vi "Main.vi"() -> ()   [LabVIEW 2020]
uses:
  <vilib>/userDefined/High Color/IMAQdx.ctl
  <vilib>/vision/Image Controls.llb/IMAQ Image.ctl
  <vilib>/DAQmx/write.llb/DAQmx Write (Analog Wfm 1Chan NSamp).vi
  <vilib>/Utility/error.llb/Error Cluster From Error Code.vi
  <vilib>/DAQmx/miscellaneous.llb/DAQmx Fill In Error Info.vi
  <vilib>/ErrorRing/Error Ring.xnode
  SuportVI2/Message Queue/Message Queue.lvlib
  SuportVI2/User Event - Stop/User Event - Stop.lvlib
  <vilib>/vision/driver/NI_Vision_Acquisition_Software.lvlib
  <vilib>/Analysis/NI_AALBase.lvlib
panel:
  in  "Generator Configuration":T1
  out "Image":T2(plugin-control)
  in  "Camera Config":cluster{"Camera Select":T3}
  in  "Exit":bool
  in  "Stop Camera":bool
  in  "Start Camera":bool
  out "Status Line":string
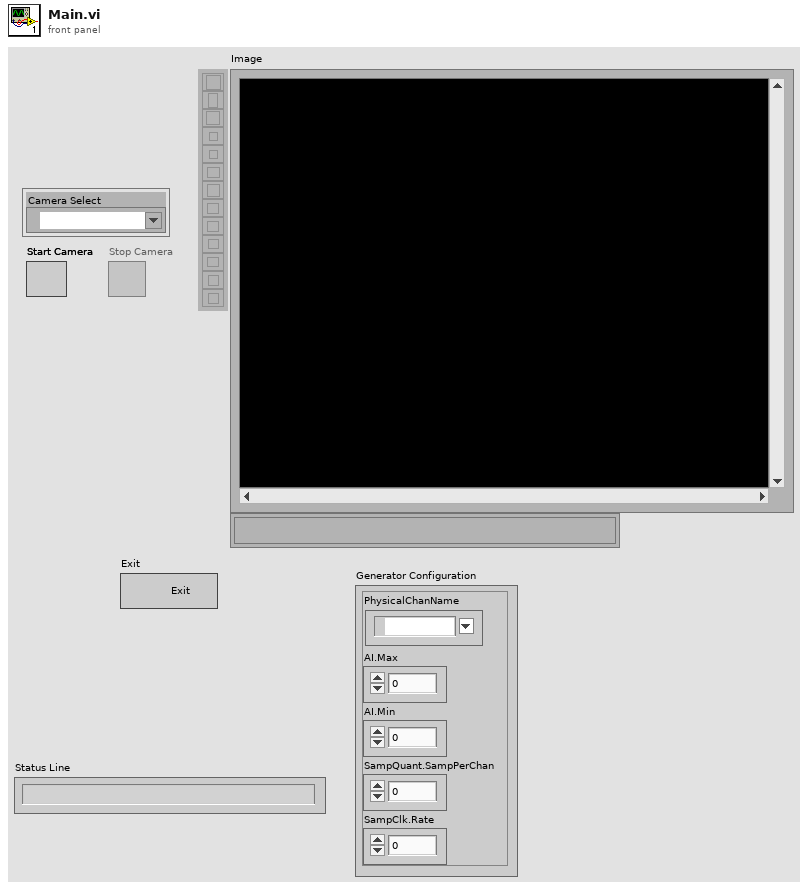
[diagram p1: front panel]
types:
  T1 = cluster{"SampClk.Rate":dbl, "SampQuant.SampPerChan":i32, "AI.Min":dbl, "AI.Max":dbl, "PhysicalChanName":tag}
  T2 = typedef "IMAQ Image.ctl" = refnum<image>
  T3 = typedef "IMAQdx.ctl" = refnum<k21>
  T4 = cluster{"DAQmx Task":refnum<k21>, "DAQmx Chanel":cluster{"SampClk.Rate":dbl, "SampQuant.SampPerChan":i32, "AI.Min":dbl, "AI.Max":dbl, "PhysicalChanName":tag}, "DB Data":dbl[][]}
  T5 = cluster{"Image":cluster{"Image original":T2, "Image copy":T2, "Image Out":T2}, "Session Config":cluster{"Session":T3}, "Data":string}
  T6 = cluster{"Start Camera":refnum<vi>, "Stop Camera":refnum<vi>, "Exit":refnum<vi>, "Camera Conf":refnum<vi>, "Status Line":refnum<vi>, "Status Line Text":string, "Camera Select":refnum<vi>}
  T7 = cluster{"UI":refnum<queue>, "Camera":refnum<queue>, "Acquire":refnum<queue>, "SinusGen":refnum<queue>}
  T8 = typedef "Image Type" = u32
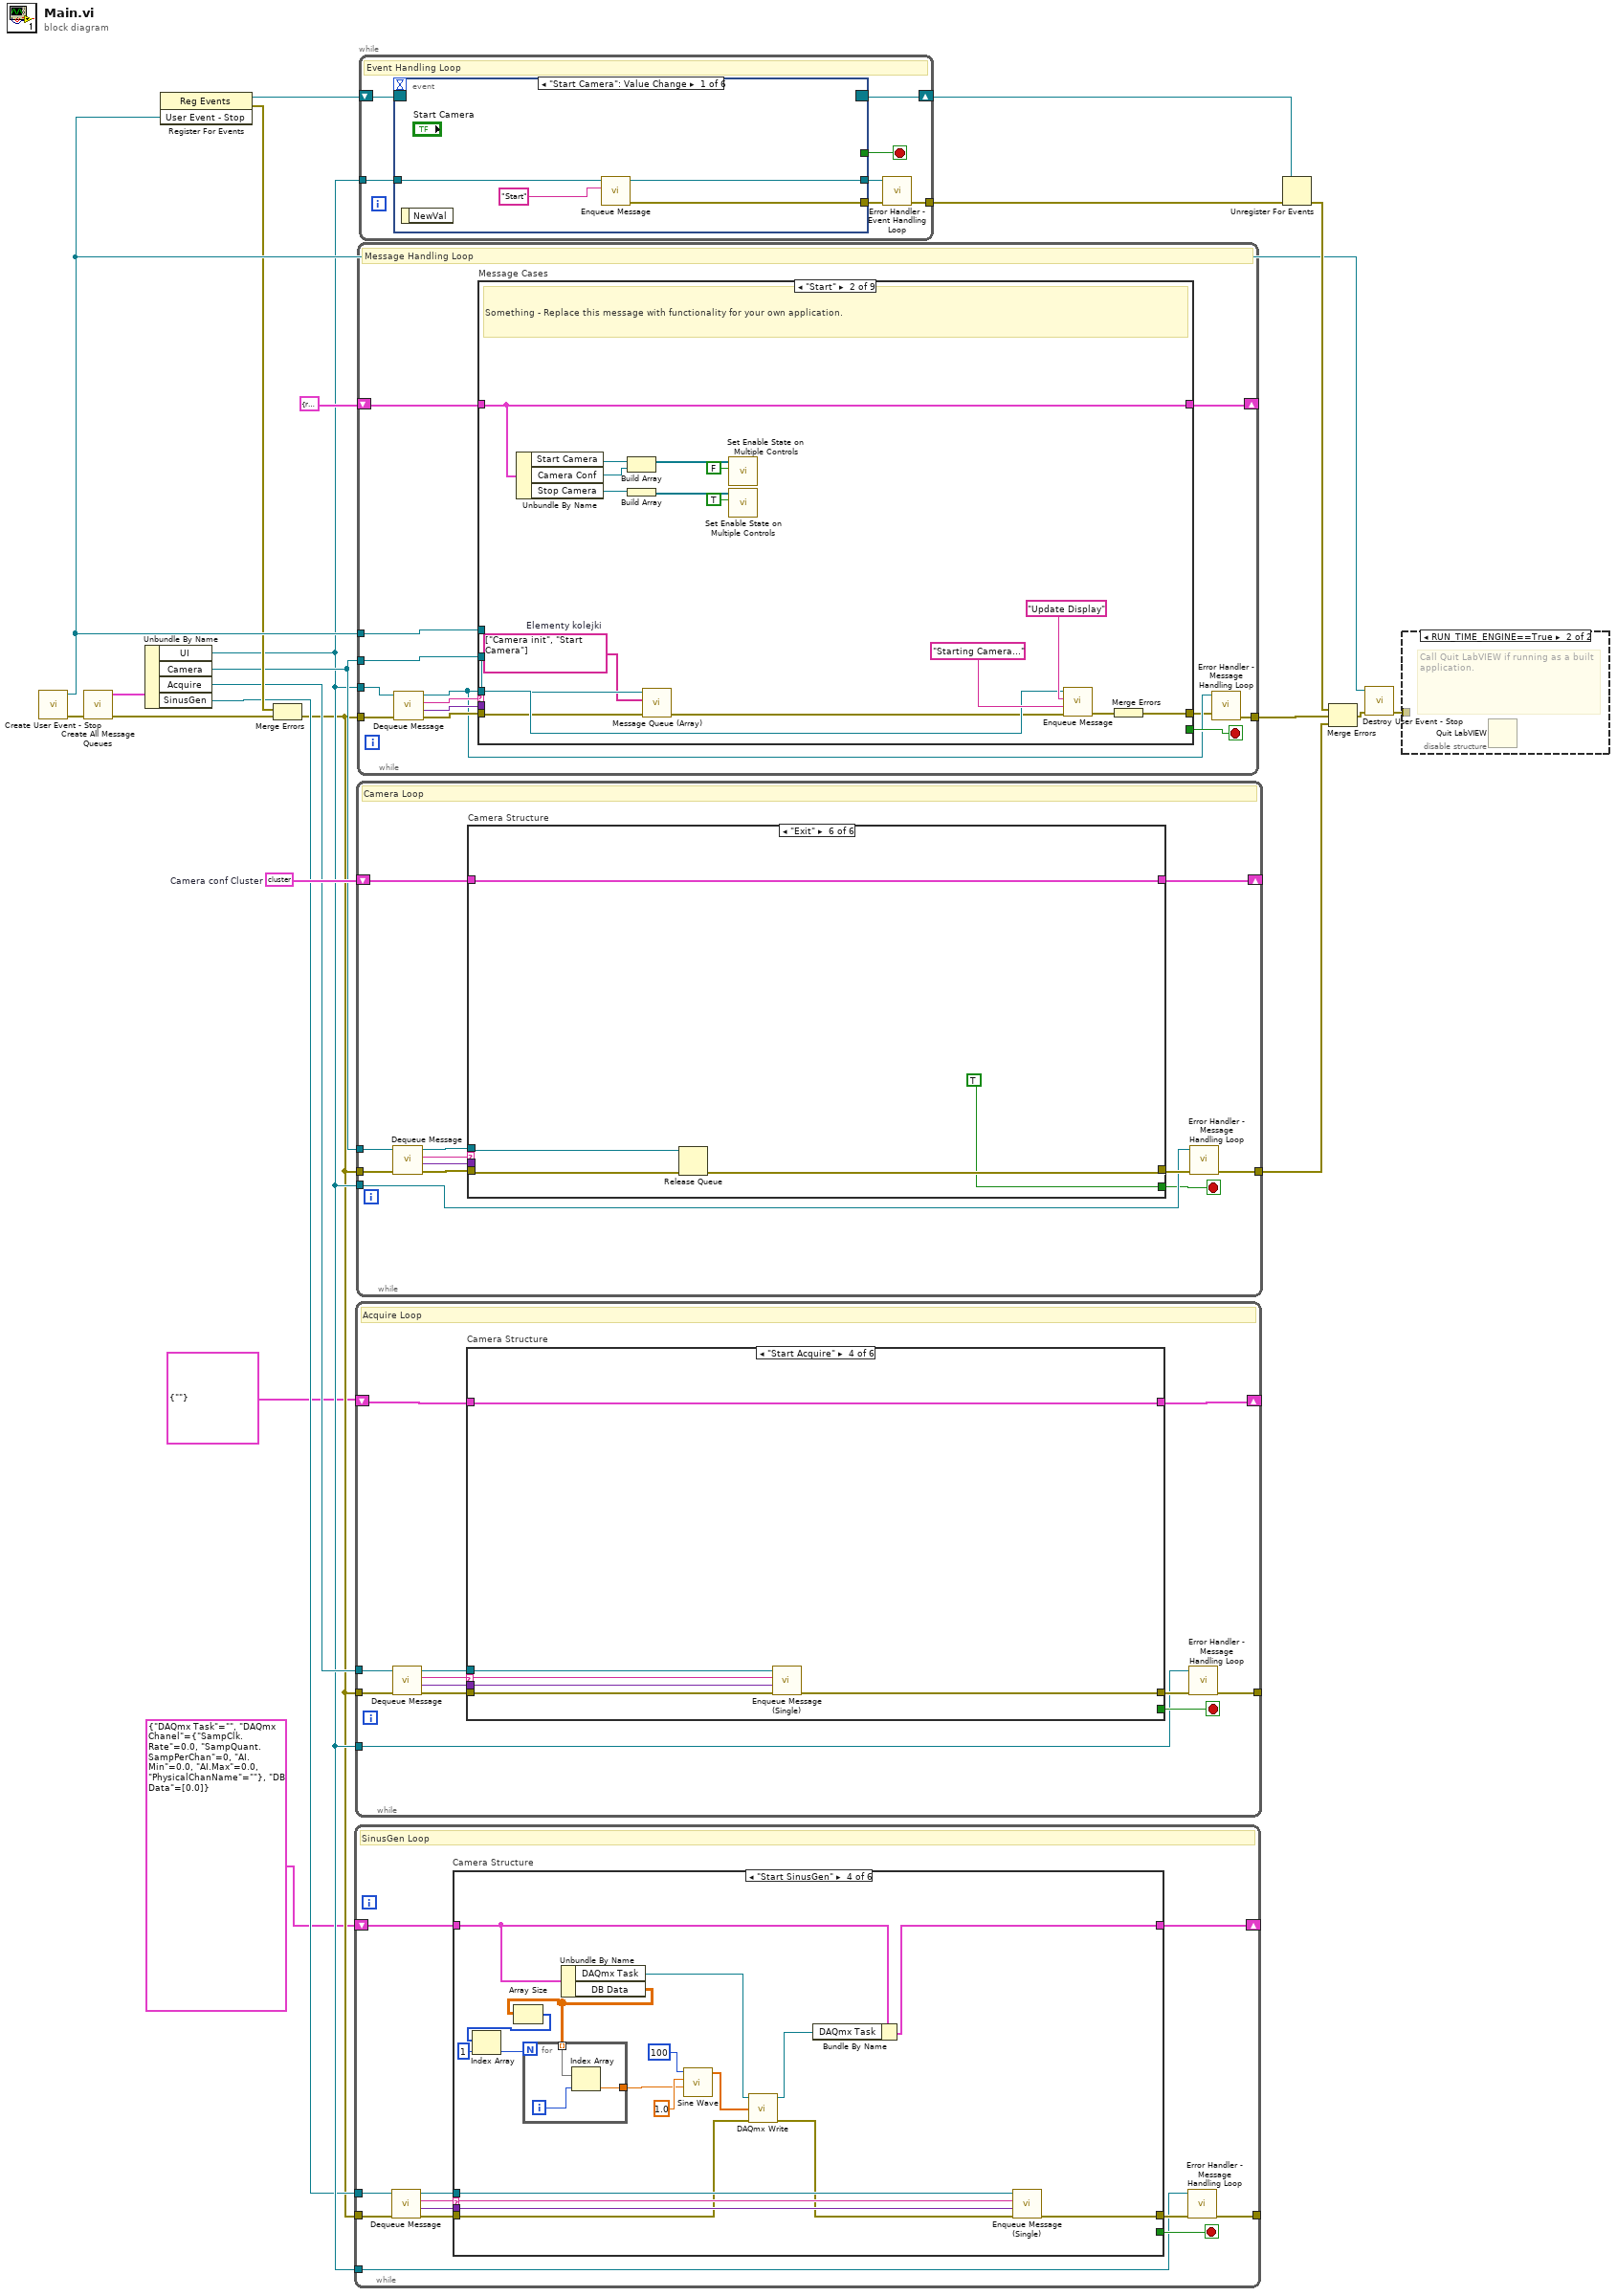
[diagram p0: block diagram]
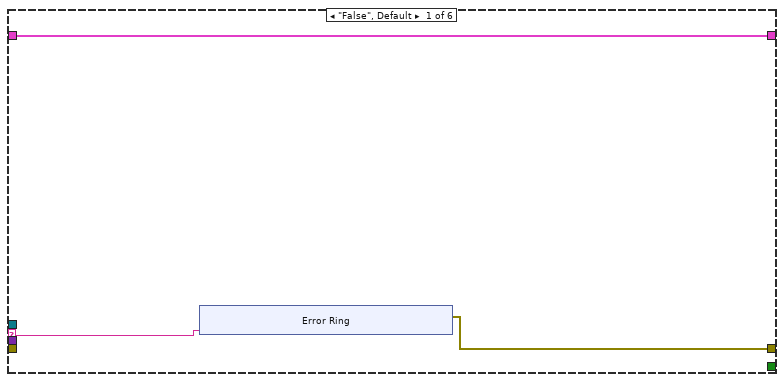
[diagram p2: hidden frame]
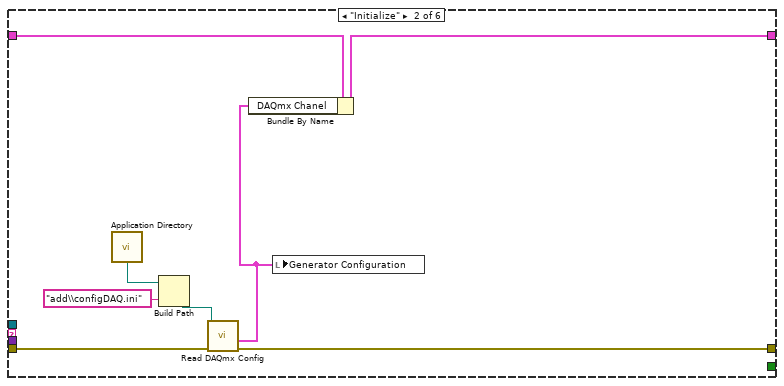
[diagram p3: hidden frame]
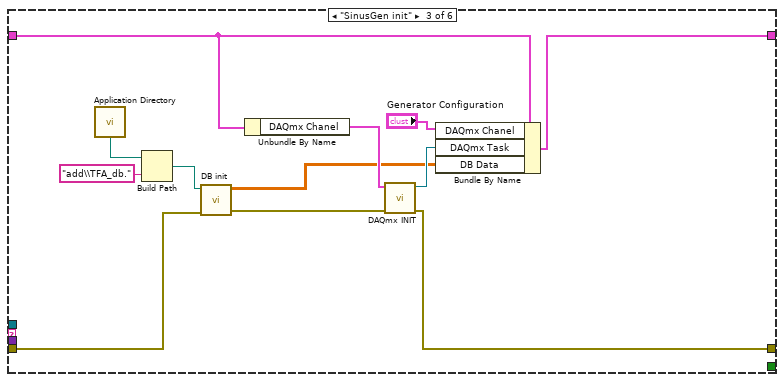
[diagram p4: hidden frame]
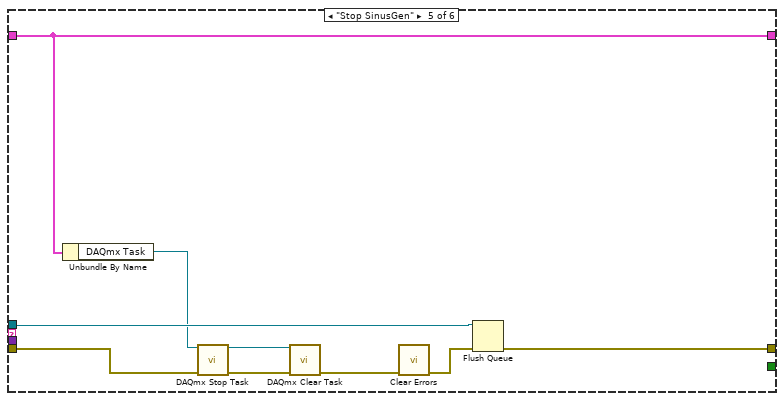
[diagram p5: hidden frame]
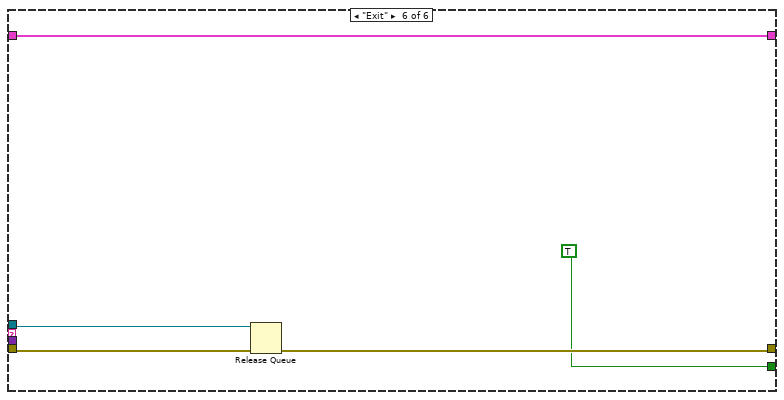
[diagram p6: hidden frame]
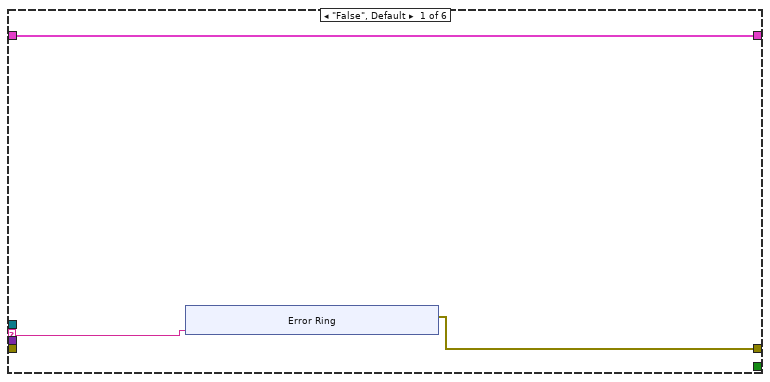
[diagram p7: hidden frame]
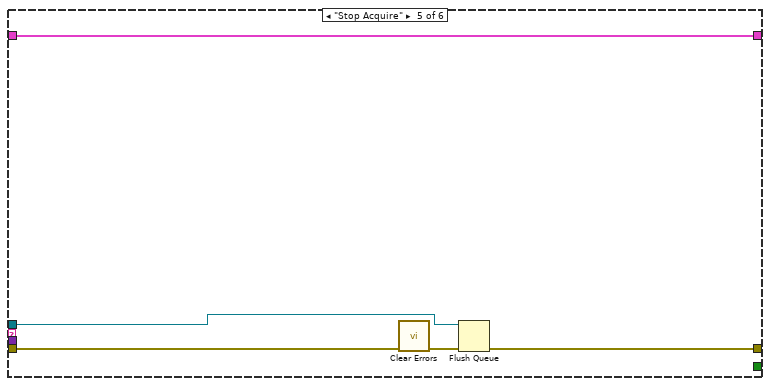
[diagram p10: hidden frame]
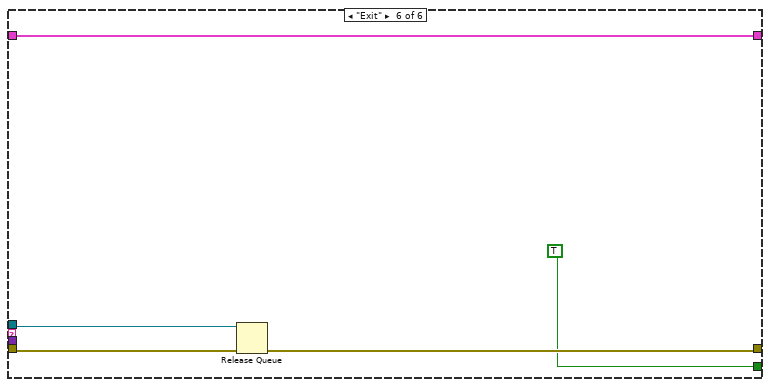
[diagram p11: hidden frame]
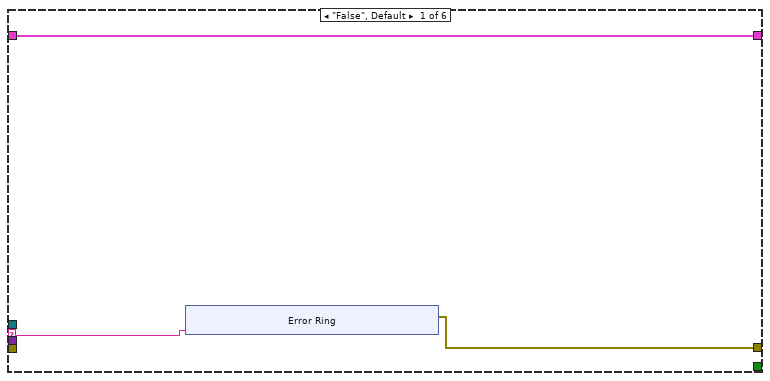
[diagram p12: hidden frame]
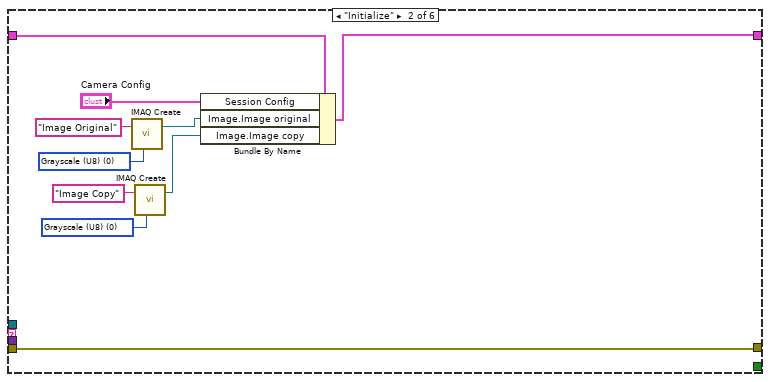
[diagram p13: hidden frame]
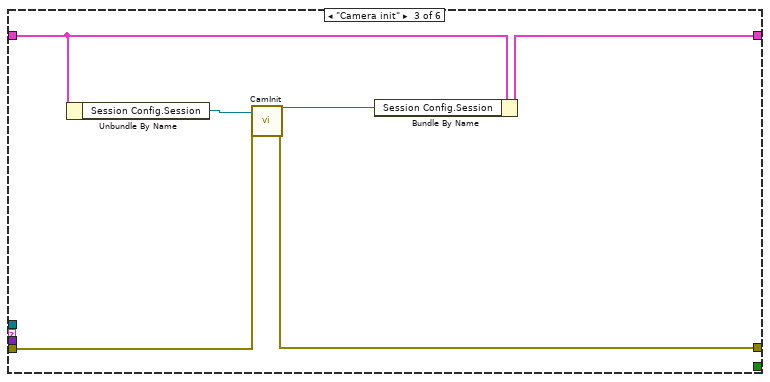
[diagram p14: hidden frame]
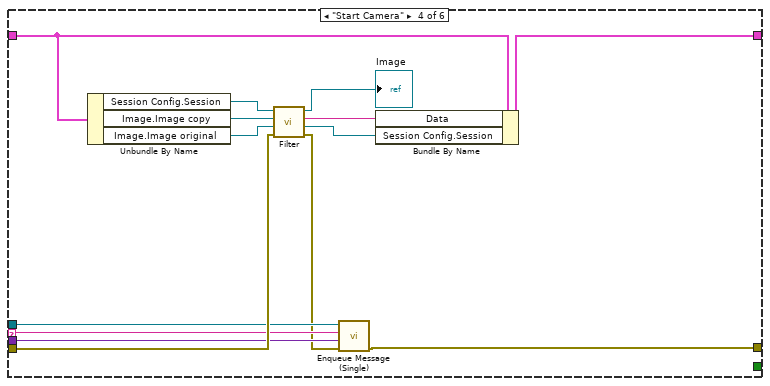
[diagram p15: hidden frame]
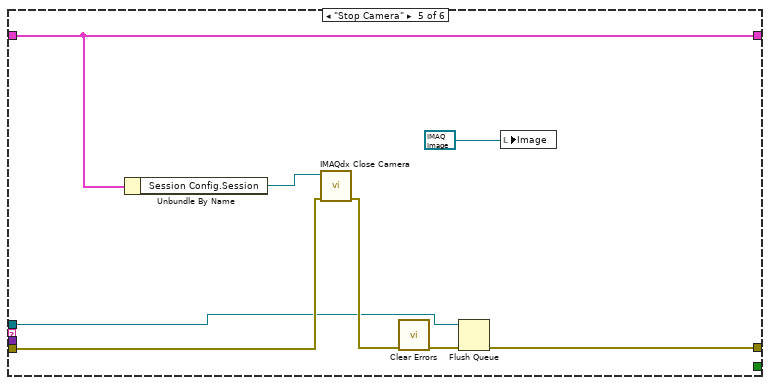
[diagram p16: hidden frame]
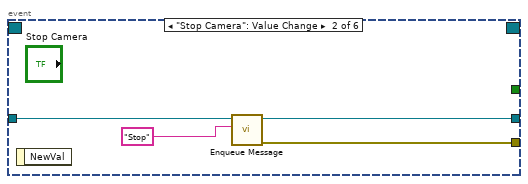
[diagram p18: hidden frame]
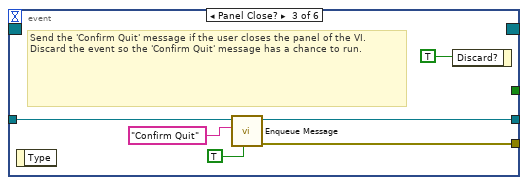
[diagram p19: hidden frame]
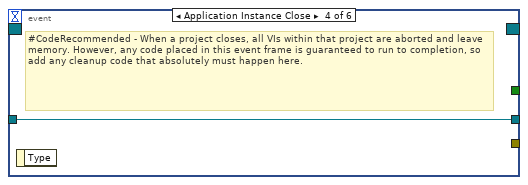
[diagram p20: hidden frame]
diagram:
  w9 = T5 {"Image"={"Image original"=refnum, "Image copy"=refnum, "Image Out"=refnum}, "Session Config"={"Session"=""}, "Data"=""}  # Camera conf Cluster
  n1 = call "Create User Event - Stop.vi"() -> ("error out"=w20:errorcluster, "User Event - Stop"=w13:refnum<user-event>)  [unwired: 10 in]
  n2 = call "Create All Message Queues.vi"("error in (no error)"=w20) -> ("error out"=w22:errorcluster, "Message Queues out"=w8:T7)  [unwired: 9 in]
  n3 = Unbundle By Name(w8) -> ("UI"=w5:refnum<queue>, "Camera"=w7:refnum<queue>, "Acquire"=w6:refnum<queue>, "SinusGen"=w4:refnum<queue>)
  n4 = register-events(w13) -> (reference out=w14:refnum<event-registration>, error out=w12:errorcluster)  [unwired: 2 in]
  n5 = Merge Errors(w12, w22) -> (w3:errorcluster)
  n6 = while {
    shift-right: [w24] -> _
    shift-left: T4 {"DAQmx Task"="", "DAQmx Chanel"={"SampClk.Rate"=0.0, "SampQuant.SampPerChan"=0, "AI.Min"=0.0, "AI.Max"=0.0, "PhysicalChanName"=""}, "DB Data"=[[0.0]]} -> [w23]
    tunnel: [w34] -> _
    tunnel: w4 -> [w31]
    tunnel: w3 -> [w26]
    tunnel: w5 -> [w25]
    stop <- w28 stop-if-true
    # "SinusGen Loop"
    n7 = call "Dequeue Message.vi"("error in (no error)"=w26, "Message Queue"=w31) -> ("error out"=w33:errorcluster, "Message Data"=w29:variant, "Message"=w27:string, "dup Message Queue"=w30:refnum<queue>)  [unwired: 6 in]
    n8 = case "Camera Structure" shown="\"Start SinusGen\"" w27 {
      selector: w27 -> [w36 _ _ w81 _ _]
      tunnel: [w37 w48 w64 w79 w93 w98] -> w32
      tunnel: w33 -> [_ w49 w59 w78 w87 w97]
      tunnel: w30 -> [_ _ _ w82 w92 w99]
      tunnel: w29 -> [_ _ _ w80 _ _]
      tunnel: [_ _ _ _ _ TRUE] -> w28
      tunnel: [w35 w46 w61 w73 w89 w95] -> w24
      tunnel: w23 -> [w35 w47 w62 w74 w89 w95]
      frame "False", Default {
        n9 = xnode "Error Ring"("parameter 0"=w36) -> ("error out"=w37:errorcluster)
      }
      frame "Initialize" {
        n10 = call <vilib>:"Application Directory.vi"() -> ("Application Directory"=w52:path)
        n11 = Build Path(base path=w52, name or relative path="add\\configDAQ.ini") -> (appended path=w50:path)
        n12 = call "Read DAQmx Config.vi"("error in (no error)"=w49, "configuration file path"=w50) -> ("error out"=w48:errorcluster, "data"=w45:T1)  [unwired: 7 in, 1 out]
        n13 = Bundle By Name(cluster=w47, "DAQmx Chanel"=w45) -> (w46:T4)
        n14 = local write "Generator Configuration"(w45) -> ()
      }
      frame "SinusGen init" {
        n15 = call <vilib>:"Application Directory.vi"() -> ("Application Directory"=w57:path)
        n16 = Build Path(base path=w57, name or relative path="add\\TFA_db.") -> (appended path=w55:path)
        n17 = call "DB init.vi"("error in (no error)"=w59, "DB path"=w55) -> ("error out"=w58:errorcluster, "DB Data"=w53:dbl[][])  [unwired: 8 in]
        n18 = Unbundle By Name(w62) -> ("DAQmx Chanel"=w63:T1)
        n19 = call "DAQmx INIT.vi"("error in"=w58, "DAQmxChannel"=w63) -> ("error out"=w64:errorcluster, "task out"=w60:refnum<k21>)  [unwired: 8 in]
        n20 = Bundle By Name(cluster=w62, "DAQmx Chanel"="Generator Configuration", "DAQmx Task"=w60, "DB Data"=w53) -> (w61:T4)
      }
      frame "Start SinusGen" {
        n21 = Unbundle By Name(w74) -> ("DAQmx Task"=w76:refnum<k21>, "DB Data"=w69:dbl[][])
        n22 = Array Size(array=w69) -> (size(s)=w67:i32[])
        n23 = Index Array(array=w67, index=1) -> (element=w68:i32)
        n24 = for {
          N: w68 -> [_]
          tunnel: w69 -> [w84] mode=indexing
          tunnel: [w83] -> w65
          i -> [w85]
          n25 = Index Array(array=w84, index=w85) -> (element=w83:dbl)
        }
        n26 = call <vilib>:"Sine Wave.vi"("samples"=100, "amplitude"=1.0, "frequency"=w65) -> ("sine wave"=w72:dbl[])  [unwired: 2 in, 2 out]
        n27 = call-poly <vilib>:"DAQmx Write.vi"("task/channels in"=w76, "data"=w72, "error in"=w78) -> ("task out"=w75:refnum<k21>, "error out"=w77:errorcluster)  [unwired: 10 in, 1 out]
        n28 = Bundle By Name(cluster=w74, "DAQmx Task"=w75) -> (w73:T4)
        n29 = call "Enqueue Message (Single).vi"("error in (no error)"=w77, "Message Data"=w80, "Message"=w81, "Message Queue"=w82) -> ("error out"=w79:errorcluster)  [unwired: 6 in, 1 out]
      }
      frame "Stop SinusGen" {
        n30 = Unbundle By Name(w89) -> ("DAQmx Task"=w88:refnum<k21>)
        n31 = call <vilib>:"DAQmx Stop Task.vi"("task/channels in"=w88, "error in"=w87) -> ("task out"=w91:refnum<k21>, "error out"=w90:errorcluster)  [unwired: 12 in]
        n32 = call <vilib>:"DAQmx Clear Task.vi"("task in"=w91, "error in"=w90) -> ("error out"=w86:errorcluster)  [unwired: 13 in]
        n33 = call <vilib>:"Clear Errors.vi"("error in (no error)"=w86) -> ("error out"=w94:errorcluster)  [unwired: 5 in, 1 out]
        n34 = Flush Queue(queue=w92, error in (no error)=w94) -> (error out=w93:errorcluster)  [unwired: 2 out]
      }
      frame "Exit" {
        n35 = Release Queue(queue=w99, error in (no error)=w97) -> (error out=w98:errorcluster)  [unwired: 1 in, 2 out]
      }
    }
    n36 = call "Error Handler - Message Handling Loop.vi"("error in (no error)"=w32, "Message Queue"=w25) -> ("dup error in"=w34:errorcluster)  [unwired: 8 in, 1 out]
  }
  n37 = while {
    shift-right: [w101] -> _
    shift-left: cluster{string} {""} -> [w100]
    tunnel: [w111] -> _
    tunnel: w6 -> [w108]
    tunnel: w3 -> [w103]
    tunnel: w5 -> [w102]
    stop <- w105 stop-if-true
    # "Acquire Loop"
    n38 = call "Dequeue Message.vi"("error in (no error)"=w103, "Message Queue"=w108) -> ("error out"=w110:errorcluster, "Message Data"=w106:variant, "Message"=w104:string, "dup Message Queue"=w107:refnum<queue>)  [unwired: 6 in]
    n39 = case "Camera Structure" shown="\"Start Acquire\"" w104 {
      selector: w104 -> [w113 _ _ w130 _ _]
      tunnel: [w114 w123 w125 w128 w135 w140] -> w109
      tunnel: w110 -> [_ w123 w125 w127 w133 w139]
      tunnel: w107 -> [_ _ _ w131 w134 w141]
      tunnel: w106 -> [_ _ _ w129 _ _]
      tunnel: [_ _ _ _ _ TRUE] -> w105
      tunnel: [w112 w122 w124 w126 w132 w137] -> w101
      tunnel: w100 -> [w112 w122 w124 w126 w132 w137]
      frame "False", Default {
        n40 = xnode "Error Ring"("parameter 0"=w113) -> ("error out"=w114:errorcluster)
      }
      frame "Initialize" {
      }
      frame "Acquire init" {
      }
      frame "Start Acquire" {
        n41 = call "Enqueue Message (Single).vi"("error in (no error)"=w127, "Message Data"=w129, "Message"=w130, "Message Queue"=w131) -> ("error out"=w128:errorcluster)  [unwired: 6 in, 1 out]
      }
      frame "Stop Acquire" {
        n42 = call <vilib>:"Clear Errors.vi"("error in (no error)"=w133) -> ("error out"=w136:errorcluster)  [unwired: 5 in, 1 out]
        n43 = Flush Queue(queue=w134, error in (no error)=w136) -> (error out=w135:errorcluster)  [unwired: 2 out]
      }
      frame "Exit" {
        n44 = Release Queue(queue=w141, error in (no error)=w139) -> (error out=w140:errorcluster)  [unwired: 1 in, 2 out]
      }
    }
    n45 = call "Error Handler - Message Handling Loop.vi"("error in (no error)"=w109, "Message Queue"=w102) -> ("dup error in"=w111:errorcluster)  [unwired: 8 in, 1 out]
  }
  n46 = while {
    shift-right: [w145] -> _
    shift-left: w9 -> [w148]
    tunnel: [w153] -> w10
    tunnel: w3 -> [w152]
    tunnel: w5 -> [w149]
    tunnel: w7 -> [w147]
    stop <- w143 stop-if-true
    # "Camera Loop"
    n47 = call "Dequeue Message.vi"("error in (no error)"=w152, "Message Queue"=w147) -> ("error out"=w151:errorcluster, "Message Data"=w144:variant, "Message"=w142:string, "dup Message Queue"=w146:refnum<queue>)  [unwired: 6 in]
    n48 = case "Camera Structure" shown="\"Exit\"" w142 {
      selector: w142 -> [w154 _ _ w184 _ _]
      tunnel: [w156 w173 w176 w181 w196 w204] -> w150
      tunnel: w151 -> [_ w173 w177 w193 w201 w203]
      tunnel: w148 -> [w155 w171 w175 w189 w200 w206]
      tunnel: w146 -> [_ _ _ w185 w195 w205]
      tunnel: [w155 w170 w174 w186 w200 w206] -> w145
      tunnel: w144 -> [_ _ _ w183 _ _]
      tunnel: [_ _ _ _ _ TRUE] -> w143
      frame "False", Default {
        n49 = xnode "Error Ring"("parameter 0"=w154) -> ("error out"=w156:errorcluster)
      }
      frame "Initialize" {
        w165 = T8 0 items=["Grayscale (U8)", "Grayscale (I16)", "Grayscale (SGL)", "Complex (CSG)", "RGB (U32)", "HSL (U32)", "RGB (U64)", "Grayscale (U16)"] ("Image Type")
        w168 = T8 0 items=["Grayscale (U8)", "Grayscale (I16)", "Grayscale (SGL)", "Complex (CSG)", "RGB (U32)", "HSL (U32)", "RGB (U64)", "Grayscale (U16)"] ("Image Type")
        n50 = call "IMAQ Create"("Image Name"="Image Original", "Image Type"=w165) -> ("New Image"=w164:T2)  [unwired: 3 in, 1 out]
        n51 = call "IMAQ Create"("Image Name"="Image Copy", "Image Type"=w168) -> ("New Image"=w167:T2)  [unwired: 3 in, 1 out]
        n52 = Bundle By Name(cluster=w171, "Session Config"="Camera Config", "Image.Image original"=w164, "Image.Image copy"=w167) -> (w170:T5)
      }
      frame "Camera init" {
        n53 = Unbundle By Name(w175) -> ("Session Config.Session"=w179:T3)
        n54 = call "CamInit.vi"("error in (no error)"=w177, "Refnum in"=w179) -> ("error out"=w176:errorcluster, "Refnum out"=w178:T3)  [unwired: 8 in]
        n55 = Bundle By Name(cluster=w175, "Session Config.Session"=w178) -> (w174:T5)
      }
      frame "Start Camera" {
        n56 = Unbundle By Name(w189) -> ("Session Config.Session"=w192:T3, "Image.Image copy"=w191:T2, "Image.Image original"=w190:T2)
        n57 = call "Filter.vi"("error in"=w193, "Image original"=w190, "Image copy"=w191, "Session Config"=w192) -> ("error out"=w182:errorcluster, "Session Out"=w187:T3, "Data"=w188:string, "Image Out"=→"Image":T2)  [unwired: 4 in]
        n58 = call "Enqueue Message (Single).vi"("error in (no error)"=w182, "Message Data"=w183, "Message"=w184, "Message Queue"=w185) -> ("error out"=w181:errorcluster)  [unwired: 6 in, 1 out]
        n59 = Bundle By Name(cluster=w189, "Data"=w188, "Session Config.Session"=w187) -> (w186:T5)
      }
      frame "Stop Camera" {
        n60 = Unbundle By Name(w200) -> ("Session Config.Session"=w199:T3)
        n61 = call <vilib>:"IMAQdx Close Camera.vi"("error in"=w201, "Session In"=w199) -> ("error out"=w197:errorcluster)  [unwired: 9 in]
        n62 = call <vilib>:"Clear Errors.vi"("error in (no error)"=w197) -> ("error out"=w198:errorcluster)  [unwired: 5 in, 1 out]
        n63 = Flush Queue(queue=w195, error in (no error)=w198) -> (error out=w196:errorcluster)  [unwired: 2 out]
        n64 = local write "Image"(T2 refnum ("Image")) -> ()
      }
      frame "Exit" {
        n65 = Release Queue(queue=w205, error in (no error)=w203) -> (error out=w204:errorcluster)  [unwired: 1 in, 2 out]
      }
    }
    n66 = call "Error Handler - Message Handling Loop.vi"("error in (no error)"=w150, "Message Queue"=w149) -> ("dup error in"=w153:errorcluster)  [unwired: 8 in, 1 out]
  }
  n67 = while {
    tunnel: w5 -> [w211]
    shift-right: [w218] -> _
    shift-left: T6 {"Start Camera"=refnum, "Stop Camera"=refnum, "Exit"=refnum, "Camera Conf"=refnum, "Status Line"=refnum, "Status Line Text"="", "Camera Select"=refnum} -> [w219]
    tunnel: w13 -> [w216]
    tunnel: w3 -> [w215]
    tunnel: [w209] -> w21
    tunnel: w7 -> [w207]
    stop <- w217 stop-if-true
    # "Message Handling Loop"
    n68 = call "Dequeue Message.vi"("error in (no error)"=w215, "Message Queue"=w211) -> ("error out"=w214:errorcluster, "Message Data"=w212:variant, "Message"=w213:string, "dup Message Queue"=w210:refnum<queue>)  [unwired: 6 in]
    n69 = case "Message Cases" shown="\"Start\"" w213 {
      selector: w213 -> [_ _ _ _ _ _ _ _ w310]
      tunnel: w210 -> [w225 w246 w266 _ _ w285 _ w309 _]
      tunnel: w214 -> [w232 w243 w263 w273 w282 w289 w292 w300 _]
      tunnel: [w233 w250 w268 w274 w276 w287 w290 w306 w311] -> w208
      tunnel: w219 -> [w231 w241 w251 w275 w281 w288 w291 w298 w312]
      tunnel: [w230 w241 w251 w275 w281 w288 w291 w298 w312] -> w218
      tunnel: [_ _ _ _ _ _ _ TRUE _] -> w217
      tunnel: w212 -> [_ _ _ w272 w280 _ _ _ _]
      tunnel: w216 -> [_ _ _ _ _ _ _ w305 _]
      tunnel: w207 -> [_ w245 w261 _ _ _ _ w303 _]
      frame "Initialize" {
        w224 = "Initialization Completed" ("Initial Message")
        # "Initialize - All initialization work should take place in this message, since other loops can potentially enqueue messages that execute immediately after this one."
        n70 = control-ref of="Start Camera"() -> (w229:refnum<vi>)
        n71 = control-ref of="Stop Camera"() -> (w220:refnum<vi>)
        n72 = control-ref of="Exit"() -> (w227:refnum<vi>)
        n73 = control-ref of="Camera Config"() -> (w223:refnum<vi>)
        n74 = control-ref of="Status Line"() -> (w228:refnum<vi>)
        n75 = Build Array(w220) -> (w221:refnum<vi>[])
        n76 = Bundle By Name(cluster=w231, "Start Camera"=w229, "Stop Camera"=w220, "Status Line"=w228, "Exit"=w227, "Status Line Text"=w224, "Camera Select"=w223) -> (w230:T6)
        n77 = call "Set Enable State on Multiple Controls.vi"("Enable?"=FALSE, "Controls"=w221) -> ()  [unwired: 10 in]
        n78 = call-poly "Enqueue Message.vi"("error in (no error)"=w232, "Message Data"=w224, "Message"="Update Display", "Message Queue"=w225) -> ("error out"=w233:errorcluster)  [unwired: 6 in, 1 out]
      }
      frame "Start" {
        w244 = string[] ["Camera init", "Start Camera"]  # Elementy kolejki
        # "Something - Replace this message with functionality for your own application."
        n79 = Unbundle By Name(w241) -> ("Start Camera"=w235:refnum<vi>, "Camera Conf"=w236:refnum<vi>, "Stop Camera"=w237:refnum<vi>)
        n80 = Build Array(w235, w236) -> (w240:refnum<vi>[])
        n81 = Build Array(w237) -> (w239:refnum<vi>[])
        n82 = call "Message Queue (Array).vi"("error in (no error)"=w243, "Message Array"=w244, "Message Queue"=w245) -> ("error out"=w242:errorcluster)  [unwired: 7 in, 1 out]
        n83 = call "Set Enable State on Multiple Controls.vi"("Enable?"=FALSE, "Controls"=w240) -> ()  [unwired: 10 in]
        n84 = call "Set Enable State on Multiple Controls.vi"("Enable?"=TRUE, "Controls"=w239) -> ()  [unwired: 10 in]
        n85 = call-poly "Enqueue Message.vi"("error in (no error)"=w242, "Message Data"="Starting Camera..." ("\"Do Something\" button pressed"), "Message"="Update Display", "Message Queue"=w246) -> ("error out"=w249:errorcluster)  [unwired: 6 in, 1 out]
        n86 = Merge Errors(w249) -> (w250:errorcluster)
      }
      frame "Stop" {
        # "Something Else - Replace this message with functionality for your own application."
        n87 = Unbundle By Name(w251) -> ("Start Camera"=w253:refnum<vi>, "Camera Conf"=w254:refnum<vi>, "Stop Camera"=w255:refnum<vi>)
        n88 = Build Array(w253, w254) -> (w258:refnum<vi>[])
        n89 = Build Array(w255) -> (w257:refnum<vi>[])
        n90 = call "Set Enable State on Multiple Controls.vi"("Enable?"=TRUE, "Controls"=w258) -> ()  [unwired: 10 in]
        n91 = call "Set Enable State on Multiple Controls.vi"("Enable?"=FALSE, "Controls"=w257) -> ()  [unwired: 10 in]
        n92 = call-poly "Enqueue Message.vi"("Priority Message? (F)"=TRUE, "error in (no error)"=w263, "Message"="Stop Camera", "Message Queue"=w261) -> ("error out"=w262:errorcluster)  [unwired: 6 in, 1 out]
        n93 = call-poly "Enqueue Message.vi"("error in (no error)"=w262, "Message Data"="Camera Stopped" ("\"Do Something Else\" button pressed"), "Message"="Update Display", "Message Queue"=w266) -> ("error out"=w267:errorcluster)  [unwired: 6 in, 1 out]
        n94 = Merge Errors(w267) -> (w268:errorcluster)
      }
      frame "Update Display" {
        # "#CodeRecommended - If you wish to decouple the Message Handling Loop from your user interface, consider creating User Events (like the \"Stop\" event in this VI) to message the Event Handling Loop whenever the user interface needs updating."
        # "Update Display - Convert the message data to a string to display in the Data Display indicator."
        n95 = Variant To Data(error in=w273, type="", Variant=w272) -> (data=→"Status Line":string, error out=w270:errorcluster)
        n96 = Merge Errors(w270) -> (w274:errorcluster)
      }
      frame "Error" {
        # "#CodeRecommended - If you ever change the name of this \"Error\" message, you'll need to update the name in the Check Loop Error.vi as well."
        # "#CodeRecommended - Consider creating a system for logging errors in some way. These errors are for notification purposes only. Handling of specific errors should be performed in the message frames that generated the error."
        # "Error - Display an error dialog. This message is sent by the \"Error Handler\" VIs at the end of other loops in this application."
        n97 = Variant To Data(error in=w282, type=errorcluster {"status"=FALSE, "code"=0, "source"=""} ("error constant"), Variant=w280) -> (data=w278:errorcluster, error out=w277:errorcluster)
        n98 = call <vilib>:"Simple Error Handler.vi"("error in (no error)"=w278) -> ()  [unwired: 4 in, 5 out]
        n99 = Merge Errors(w277) -> (w276:errorcluster)
      }
      frame "Confirm Quit" {
        # "#CodeNeeded - If you want to provide an \"Are you sure\" dialog (or some other notification) before the application exits, place that code here. This message is typically sent from a Panel Close? event."
        # "Confirm Quit - Message that can confirm whether or not the user wants to exit the application."
        n100 = call-poly "Enqueue Message.vi"("Priority Message? (F)"=TRUE, "error in (no error)"=w289, "Message"="Exit", "Message Queue"=w285) -> ("error out"=w286:errorcluster)  [unwired: 6 in, 1 out]
        n101 = Merge Errors(w286) -> (w287:errorcluster)
      }
      frame "---Copy This Frame---" {
        # "Duplicate this frame when creating new messages.  Change this comment in the duplicated frame to describe this message."
        n102 = Merge Errors(w292) -> (w290:errorcluster)
      }
      frame "Exit" {
        # "Stop the VI"
        # "Exit - Exit the application."
        n103 = call "Enqueue Message (Single).vi"("Priority Message? (F)"=TRUE, "error in (no error)"=w300, "Message"="Exit", "Message Queue"=w303) -> ("error out"=w299:errorcluster)  [unwired: 6 in, 1 out]
        n104 = Unbundle By Name(w298) -> ("Start Camera"=w295:refnum<vi>, "Stop Camera"=w294:refnum<vi>, "Camera Conf"=w293:refnum<vi>)
        n105 = call "Fire User Event - Stop.vi"("User Event - Stop"=w305) -> ("error out"=w304:errorcluster)  [unwired: 10 in]
        n106 = Release Queue(queue=w309, error in (no error)=w299) -> (error out=w307:errorcluster)  [unwired: 1 in, 2 out]
        n107 = Build Array(w295, w294, w293) -> (w296:refnum<vi>[])
        n108 = Merge Errors(w304, w307) -> (w306:errorcluster)
        n109 = call "Set Enable State on Multiple Controls.vi"("Enable?"=TRUE, "Controls"=w296) -> ()  [unwired: 10 in]
      }
      frame Default {
        # "'Default' case only runs if there is a message that isn't defined in any of the other cases.  Output a programming error."
        n110 = xnode "Error Ring"("parameter 0"=w310) -> ("error out"=w311:errorcluster)
      }
    }
    n111 = call "Error Handler - Message Handling Loop.vi"("error in (no error)"=w208, "Message Queue"=w210) -> ("dup error in"=w209:errorcluster)  [unwired: 8 in, 1 out]
  }
  n112 = while {
    tunnel: w5 -> [w326]
    shift-right: [w324] -> w17
    shift-left: w14 -> [w325]
    tunnel: [w320] -> w15
    stop <- w322 stop-if-true
    # "Event Handling Loop"
    n113 = event shown="[0] \"Start Camera\": Value Change" {
      selector: w325 -> [_ _ _ _ _ _]
      dyn-events: [_ _ _ _ _ _] -> w324
      timeout: _ -> [_ _ _ _ _ _]
      tunnel: [_ _ _ _ _ TRUE ("Discard?")] -> w322
      tunnel: w326 -> [w330 w334 w339 w341 w346 w349]
      tunnel: [w327 w331 w338 _ w345 _] -> w323
      tunnel: [w329 w333 w337 w341 w344 w349] -> w321
      event "Start Camera": Value Change {
        n114 = event-data() -> ()  [unwired: 1 in, 1 out]
        n115 = call-poly "Enqueue Message.vi"("Message"="Start", "Message Queue"=w330) -> ("error out"=w327:errorcluster, "dup Message Queue"=w329:refnum<queue>)  [unwired: 8 in]
      }
      event "Stop Camera": Value Change {
        n116 = event-data() -> ()  [unwired: 1 in, 1 out]
        n117 = call-poly "Enqueue Message.vi"("Message"="Stop", "Message Queue"=w334) -> ("error out"=w331:errorcluster, "dup Message Queue"=w333:refnum<queue>)  [unwired: 8 in]
      }
      event Panel Close? {
        # "Send the 'Confirm Quit' message if the user closes the panel of the VI. Discard the event so the 'Confirm Quit' message has a chance to run."
        n118 = event-data() -> ()  [unwired: 1 in, 1 out]
        n119 = call-poly "Enqueue Message.vi"("Priority Message? (F)"=TRUE, "Message"="Confirm Quit", "Message Queue"=w339) -> ("error out"=w338:errorcluster, "dup Message Queue"=w337:refnum<queue>)  [unwired: 7 in]
        n120 = event-data("Discard?"=TRUE) -> ()  [unwired: 1 in, 1 out]
      }
      event Application Instance Close {
        # "#CodeRecommended - When a project closes, all VIs within that project are aborted and leave memory. However, any code placed in this event frame is guaranteed to run to completion, so add any cleanup code that absolutely must happen here."
        n121 = event-data() -> ()  [unwired: 1 in, 1 out]
      }
      event "Exit": Value Change {
        n122 = event-data() -> ()  [unwired: 1 in, 1 out]
        n123 = call-poly "Enqueue Message.vi"("Priority Message? (F)"=TRUE, "Message"="Exit", "Message Queue"=w346) -> ("error out"=w345:errorcluster, "dup Message Queue"=w344:refnum<queue>)  [unwired: 7 in]
      }
      event User Event {
        # "The Message Handling Loop processed an \"Exit\" message, which fired this event to stop the Event Handling Loop."
        n124 = event-data() -> ()  [unwired: 1 in, 1 out]
        n125 = local write "Status Line"("Exiting application" ("VI Stopped")) -> ()
      }
    }
    n126 = call "Error Handler - Event Handling Loop.vi"("error in (no error)"=w323, "Message Queue"=w321) -> ("dup error in"=w320:errorcluster)  [unwired: 8 in, 1 out]
  }
  n127 = Unregister For Events(event registration refnum=w17, error in=w15) -> (error out=w18:errorcluster)
  n128 = Merge Errors(w18, w21, w10) -> (w19:errorcluster)
  n129 = call "Destroy User Event - Stop.vi"("error in (no error)"=w19, "User Event - Stop"=w13) -> ("error out"=w16:errorcluster)  [unwired: 9 in]
  n130 = disable-structure shown="RUN_TIME_ENGINE==True" {
    disable-tunnel: w16 -> [_ _]
    frame condition #0 (active) {
    }
    frame condition #1 {
      # "Call Quit LabVIEW if running as a built application."
      n131 = Quit LabVIEW() -> ()  [unwired: 1 in]
    }
  }
